vi "convert_value.vi"(8 "error in (no error)":errorcluster, 10 "value in":string, 11 "PrepLineObject in":refnum<class "PrepLineObject.lvclass">) -> (0 "error out":errorcluster, 2 "converted value out":string, 3 "PrepLineObject out":refnum<class "PrepLineObject.lvclass">)   [LabVIEW 2017, in "PrepLineObject.lvclass"]
doc: "converts the input value according to the conversion formula (private property inside the VI)"
uses:
  PrepLineObject.lvclass
  <vilib>/gmath/NI_Gmath.lvlib
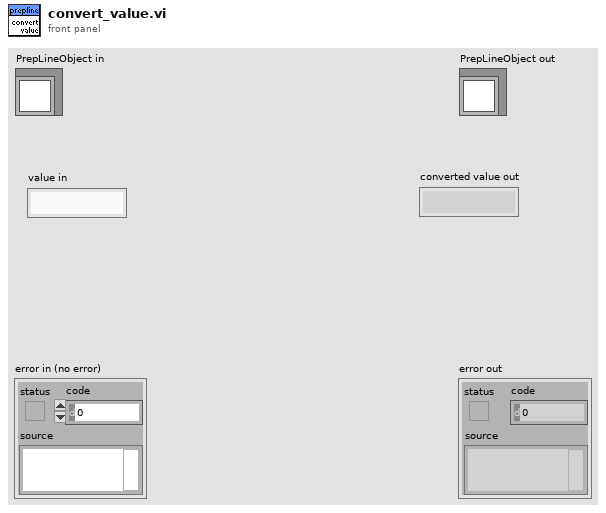
[diagram p1: front panel]
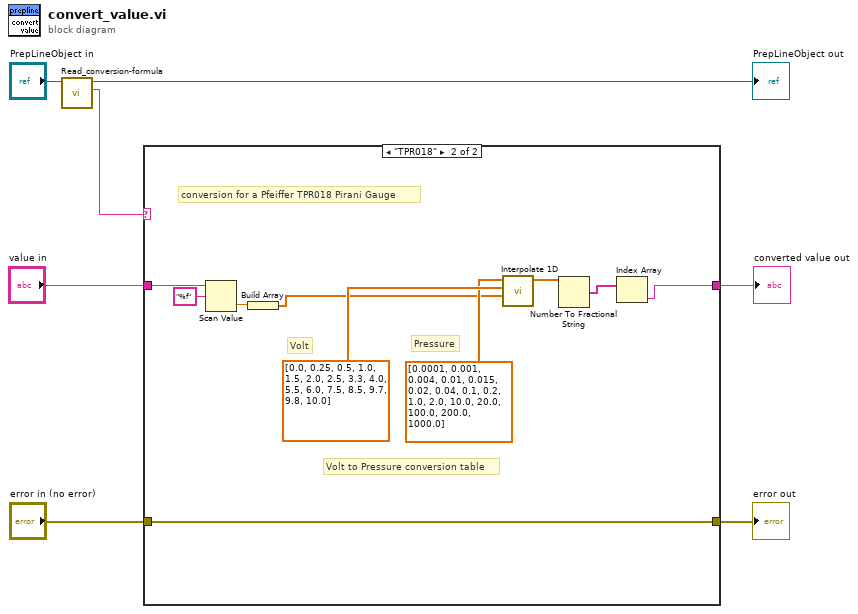
[diagram p0: block diagram]
diagram:
  n1 = call-dynamic "Read_conversion-formula.vi"("PrepLineObject in"="PrepLineObject in") -> ("conversion formula"=w5:string, "PrepLineObject out"=→"PrepLineObject out":refnum<class "PrepLineObject.lvclass">)  [unwired: 8 in, 1 out]
  n2 = case shown="\"TPR018\"" w5 {
    tunnel: "value in" -> [w9 w17]
    tunnel: [w9 w11] -> w3
    tunnel: "error in (no error)" -> [w8 w10]
    tunnel: [w8 w10] -> w1
    frame "False", Default {
    }
    frame "TPR018" {
      # "Volt to Pressure conversion table"
      # "Pressure"
      # "Volt"
      # "conversion for a Pfeiffer TPR018 Pirani Gauge"
      n3 = Scan Value(string=w17, format string="%f") -> (value=w15:dbl)  [unwired: 1 in, 1 out]
      n4 = Build Array(w15) -> (w14:dbl[])
      n5 = call <vilib>:"Interpolate 1D.vi"("xi"=w14, "X"=dbl[] [0.0, 0.25, 0.5, 1.0, 1.5, 2.0, 2.5, 3.3, 4.0, 5.5, 6.0, 7.5, 8.5, 9.7, 9.8, 10.0] ("Y"), "Y"=dbl[] [0.0001, 0.001, 0.004, 0.01, 0.015, 0.02, 0.04, 0.1, 0.2, 1.0, 2.0, 10.0, 20.0, 100.0, 200.0, 1000.0]) -> ("yi"=w13:dbl[])  [unwired: 6 in, 2 out]
      n6 = Number To Fractional String(number=w13) -> (F-format string=w12:string[])  [unwired: 3 in]
      n7 = Index Array(array=w12) -> (element=w11:string)  [unwired: 1 in]
    }
  }
  "error out" <- w1
  "converted value out" <- w3
